vi "Write nextInChain.vi"(8 "error in (no error)":errorcluster, 10 "Chain.lvclass":refnum<class "Chain.lvclass">, 11 "Add in":refnum<class "Add.lvclass">) -> (0 "error out":errorcluster, 3 "Add out":refnum<class "Add.lvclass">)   [LabVIEW 2018, in "Add.lvclass"]
uses:
  Add.lvclass
  Chain Class/Chain.lvclass
  Add.lvclass/Add.ctl
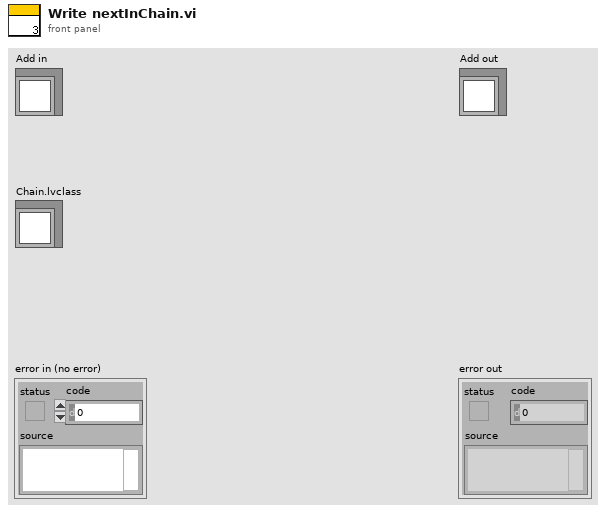
[diagram p1: front panel]
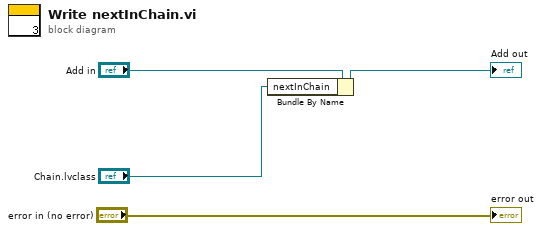
[diagram p0: block diagram]
diagram:
  n1 = Bundle By Name(cluster="Add in", "nextInChain"="Chain.lvclass") -> (→"Add out":refnum<class "Add.lvclass">)
  "error out" <- "error in (no error)"
